vi "Start Tovey Receive.vi"(8 "error in (no error)":errorcluster, 11 "Model in":refnum<class "Model.lvclass">) -> (0 "error out":errorcluster, 3 "Model out":refnum<class "Model.lvclass">)   [LabVIEW 2015, in "Model.lvclass"]
uses:
  Model.lvclass
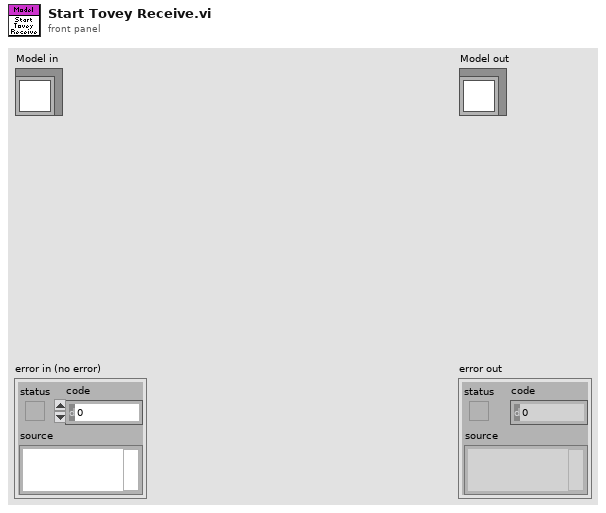
[diagram p1: front panel]
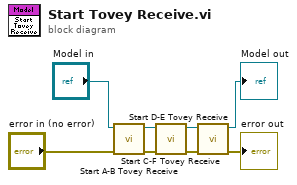
[diagram p0: block diagram]
diagram:
  n1 = call "Start A-B Tovey Receive.vi"("error in (no error)"="error in (no error)", "Model in"="Model in") -> ("error out"=w3:errorcluster, "Model out"=w7:refnum<class "Model.lvclass">)  [unwired: 8 in]
  n2 = call "Start C-F Tovey Receive.vi"("error in (no error)"=w3, "Model in"=w7) -> ("error out"=w2:errorcluster, "Model out"=w6:refnum<class "Model.lvclass">)  [unwired: 8 in]
  n3 = call "Start D-E Tovey Receive.vi"("error in (no error)"=w2, "Model in"=w6) -> ("error out"=→"error out":errorcluster, "Model out"=→"Model out":refnum<class "Model.lvclass">)  [unwired: 8 in]
